vi "zadanie_1.vi"() -> ()   [LabVIEW 2017]
panel:
  in  "zatrzymaj program":bool
  out "zmieniony tekst":string
  in  "wprowadz tekst":string
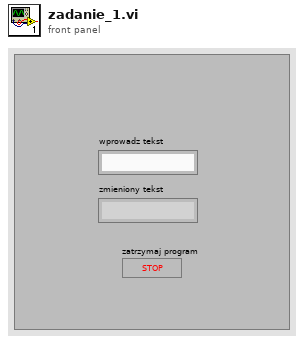
[diagram p1: front panel]
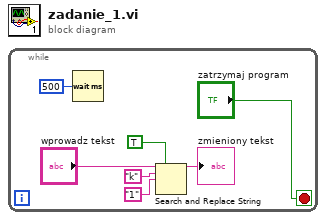
[diagram p0: block diagram]
diagram:
  n1 = while {
    stop <- "zatrzymaj program" stop-if-true
    n2 = Wait (ms)(milliseconds to wait=u32 500) -> ()  [unwired: 1 out]
    n3 = Search and Replace String(replace all?=TRUE ("replace all? (F)"), input string="wprowadz tekst", search string="k", replace string="1") -> (result string=→"zmieniony tekst":string)  [unwired: 4 in, 3 out]
  }
